vi "Proccess Async Lockin Channel.vi"(4 "Lock-in settings":T1={"Averaging period, s"=0.0, "Output Representation"=enum."Real/Imaginary", "Output value"=enum."RMS", "Phase delay, points"=0} {"Averaging period, s" format="%#_6p"}, 5 "Channel info":T2, 6 "Overwrite\nclock, Hz":dbl, 7 "Raw chunk size":i64, 8 "error in (no error)":errorcluster, 9 "Settings":string, 10 "group name":string, 11 "Data file path":path) -> (0 "error out":errorcluster, 1 "Settings out":string, 2 "Channel Length":u64, 3 "signal(s) out":waveform(dbl)[](array[waveform]))   [LabVIEW 2016]
uses:
  CH_name_pts_phase.ctl
  Syncronous Lockin Settings.ctl
  Utilities/Replace dt SGL.vi
  <vilib>/Waveform/WDTOps.llb/WDT Append Waveforms DBL.vi
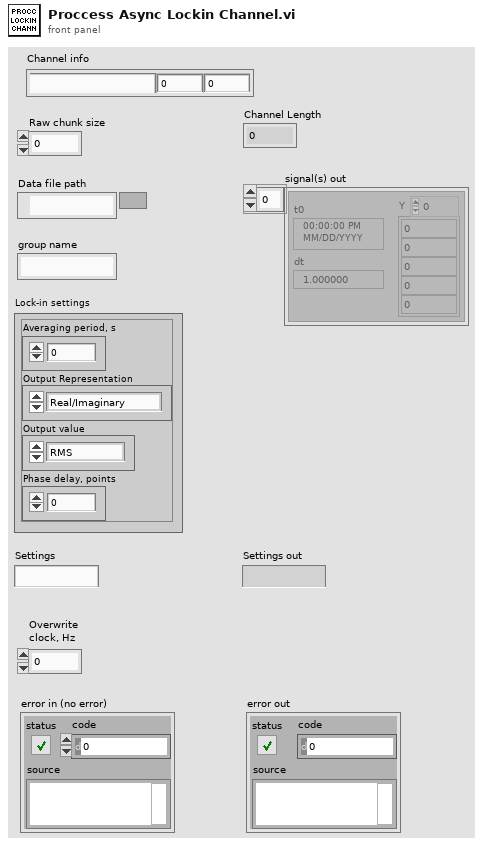
[diagram p1: front panel]
types:
  T1 = typedef "Syncronous Lockin Settings.ctl" = cluster{"Averaging period, s":dbl, "Output Representation":enum16{"Real/Imaginary", "Polar"}, "Output value":enum16{"Amplitude", "RMS", "Peak-to-Peak"}, "Phase delay, points":i32}
  T2 = typedef "CH_name_pts_phase.ctl" = cluster{"Channel":string, "pts per sine wave":i32, "Phase":dbl}
  T3 = enum16{"open", "open or create", "create or replace", "create", "open (read-only)"}
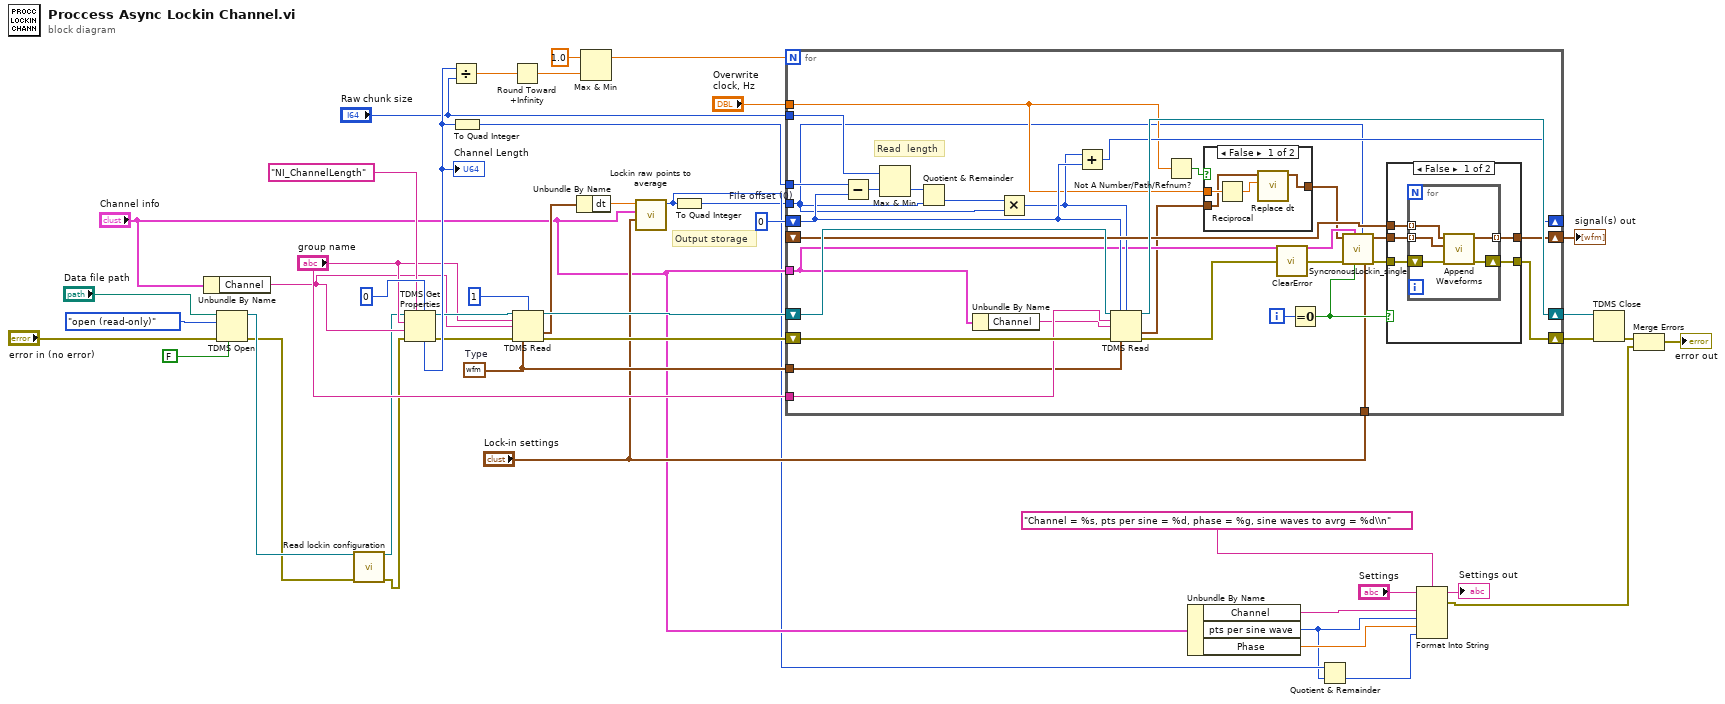
[diagram p0: block diagram]
diagram:
  w23 = waveform(sgl) {"t0"=timestamp(0 s since 1904-01-01), "dt"=1.0, "Y"=[]}  # Type
  w35 = i64 0  # File offset (0)
  # "Output storage"
  n1 = Unbundle By Name("Channel info") -> ("Channel"=w24:string)
  n2 = TDMS Open(6:FALSE ("disable buffering (T)"), 8:"error in (no error)", 10:T3."open (read-only)" ("TDMS open mode"), 11:"Data file path") -> (0:w3:errorcluster, 3:w5:refnum<k34>)  [unwired: 3 in]
  n3 = call "Read lockin configuration.vi"("tdms file"=w5, "Error In"=w3) -> ("tdms file out"=w4:refnum<k34>, "Error Out"=w2:errorcluster)  [unwired: 6 in, 6 out]
  n4 = TDMS Get Properties(5:u64 0, 7:"NI_ChannelLength" ("property name"), 8:w2, 9:w24, 10:"group name", 11:w4) -> (0:w29:errorcluster, 3:w27:refnum<k34>, 4:w41:u64)  [unwired: 3 out]
  "Channel Length" <- w41
  n5 = Divide(x=w41, y="Raw chunk size") -> (x/y=w33:dbl)
  n6 = To Quad Integer(1:w41) -> (0:w42:i64)
  n7 = Round Toward +Infinity(x=w33) -> (ceil(x): smallest int >= x=w34:dbl)
  n8 = TDMS Read(0:w27, 2:i64 1 ("count (-1: all)"), 5:"group name", 7:w24, 11:w29, 12:w23) -> (4:w26:refnum<k34>, 10:w21:waveform(sgl), 15:w28:errorcluster)  [unwired: 2 in, 3 out]
  n9 = Unbundle By Name(w21) -> ("dt"=w20:dbl)
  n10 = Max & Min(x=1.0, y=w34) -> (max(x,y)=w39:dbl)  [unwired: 1 out]
  n11 = call "Lockin raw points to average.vi"("Lock-in settings"="Lock-in settings", "CH name                          points   phase"="Channel info", "dt"=w20) -> ("Lockin raw points to average"=w7:i32)  [unwired: 8 in]
  n12 = To Quad Integer(1:w7) -> (0:w1:i64)
  n13 = for {
    N: w39 -> [_]
    shift-right: [w63] -> w18
    shift-left: w28 -> [w76]
    shift-right: [w73] -> w37
    shift-left: w26 -> [w75]
    tunnel: "group name" -> [w74]
    tunnel: "Channel info" -> [w52]
    shift-right: [w72] -> _
    shift-left: w35 -> [w62]
    tunnel: "Raw chunk size" -> [w56]
    tunnel: w23 -> [w71]
    shift-right: [w68] -> w45
    shift-left: _ -> [w67]
    tunnel: w1 -> [w48]
    tunnel: w42 -> [w57]
    tunnel: "Overwrite\nclock, Hz" -> [w55]
    tunnel: "Lock-in settings" -> [w47]
    i -> [w69]
    # "Read  length"
    n14 = Subtract(x=w57, y=w62) -> (x-y=w61:i64)
    n15 = Max & Min(x=w56, y=w61) -> (min(x,y)=w60:i64)  [unwired: 1 out]
    n16 = Quotient & Remainder(x=w60, y=w48) -> (floor(x/y)=w59:i64)  [unwired: 1 out]
    n17 = Unbundle By Name(w52) -> ("Channel"=w53:string)
    n18 = Multiply(x=w59, y=w48) -> (x*y=w58:i64)
    n19 = Add(x=w58, y=w62) -> (x+y=w72:i64)
    n20 = TDMS Read(0:w75, 1:w62, 2:w58, 5:w74, 7:w53, 11:w76, 12:w71) -> (4:w73:refnum<k34>, 10:w50:waveform(sgl), 15:w54:errorcluster)  [unwired: 1 in, 3 out]
    n21 = Not A Number/Path/Refnum?(number/path/refnum=w55) -> (NaN/Path/Refnum?=w51:bool)
    n22 = case shown="False" w51 {
      tunnel: w50 -> [w78 w81]
      tunnel: [w80 w81] -> w49
      tunnel: w55 -> [w79 _]
      frame False {
        n23 = Reciprocal(x=w79) -> (1/x=w77:dbl)
        n24 = call-poly "Replace dt.vi"("dt"=w77, "Waveform in"=w78) -> ("Waveform out"=w80:waveform(sgl))  [unwired: 9 in]
      }
      frame True {
      }
    }
    n25 = call <vilib>:"ClearError.vi"("error in (no error)"=w54) -> ("error out"=w70:errorcluster)
    n26 = Equal To 0?(x=w69) -> (x = 0?=w66:bool)
    n27 = call "SyncronousLockin_single.vi"("Lock-in settings"=w47, "Raw points to average"=w48, "First chunk?"=w66, "CH name                          points   phase"=w52, "error in (no error)"=w70, "Data"=w49) -> ("error out"=w65:errorcluster, "signal(s) out"=w64:waveform(dbl)[])  [unwired: 4 in]
    n28 = case shown="False" w66 {
      tunnel: [w86 w93] -> w68
      tunnel: w67 -> [w84 _]
      tunnel: w65 -> [w85 w92]
      tunnel: w64 -> [w83 w93]
      tunnel: [w82 w92] -> w63
      frame False {
        n29 = for {
          tunnel: [w91] -> w86 mode=indexing
          tunnel: w84 -> [w90] mode=indexing
          shift-right: [w88] -> w82
          shift-left: w85 -> [w89]
          tunnel: w83 -> [w87] mode=indexing
          n30 = call-poly <vilib>:"Append Waveforms.vi"("error in (no error)"=w89, "waveform B"=w87, "waveform A"=w90) -> ("error out"=w88:errorcluster, "waveform out"=w91:waveform(dbl))  [unwired: 7 out]
        }
      }
      frame True {
      }
    }
  }
  "signal(s) out" <- w45
  n31 = Unbundle By Name("Channel info") -> ("Channel"=w14:string, "pts per sine wave"=w6:i32, "Phase"=w13:dbl)
  n32 = Quotient & Remainder(x=w7, y=w6) -> (floor(x/y)=w8:i32)  [unwired: 1 out]
  n33 = Format Into String(format string="Channel = %s, pts per sine = %d, phase = %g, sine waves to avrg = %d\\n", initial string="Settings", w14, w6, w13, w8) -> (resulting string=→"Settings out":string, error out=w9:errorcluster)  [unwired: 1 in]
  n34 = TDMS Close(8:w18, 11:w37) -> (0:w17:errorcluster)  [unwired: 1 out]
  n35 = Merge Errors(w17, w9) -> (→"error out":errorcluster)
